vi "spy shoot up.vi"(0 "RPM setting":dbl) -> ()   [LabVIEW 2015]
uses:
  <vilib>/Rock Robotics/WPI/Solenoid/WPI_SolenoidValue.ctl
  <vilib>/Rock Robotics/WPI/CAN/TalonSRX/WPI_CANTalonSRX_APIControlMode.ctl
  <vilib>/Rock Robotics/WPI/Solenoid/WPI_SolenoidSetEnum.vi
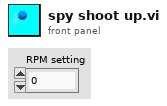
[diagram p1: front panel]
types:
  T1 = typedef "WPI_SolenoidDevRef.ctl" = cluster{"DevStatus":errorcluster, "Pneumatics Control Module":u8, "Forward Solenoid Channel":T2, "Reverse Solenoid Channel":T2}
  T2 = typedef "WPI_SolenoidChannel.ctl" = enum8{"Solenoid 0", "Solenoid 1", "Solenoid 2", "Solenoid 3", "Solenoid 4", "Solenoid 5", "Solenoid 6", "Solenoid 7", "Invalid"}
  T3 = typedef "WPI_MotorControlDeviceRef.ctl" = cluster{"DeviceStatus":errorcluster, "Type":T4, "PWM":cluster{"PWM Channel":T5, "DeadBand":T6}, "CAN":cluster{"Device Number":u8, "Control Mode":T7, "Semaphore":T8, "Max Vout":dbl, "TalonSRX Control Mode":T9}, "Invert":bool}
  T4 = typedef "WPI_MotorControlType.ctl" = enum16{"PWM", "CAN", "CANTalonSRX"}
  T5 = typedef "FPGA_DIOPWMChannel.ctl" = enum8{"PWM 0", "PWM 1", "PWM 2", "PWM 3", "PWM 4", "PWM 5", "PWM 6", "PWM 7", "PWM 8", "PWM 9", "PWM MXP 0", "PWM MXP 1", "PWM MXP 2", "PWM MXP 3", "PWM MXP 4", "PWM MXP 5", "PWM MXP 6", "PWM MXP 7", "PWM MXP 8", "PWM MXP 9", "Invalid"}
  T6 = typedef "WPI_PWMDeadband.ctl" = cluster{"Name":string, "maxPositivePwm":i32, "minPositivePwm":i32, "centerPwm":i32, "maxNegativePwm":i32, "minNegativePwm":i32, "angularRange":u16}
  T7 = typedef "WPI_CANJaguar_ControlMode.ctl" = enum8{"Percent VBus", "Current", "Speed", "Position", "Voltage"}
  T8 = typedef "Semaphore RefNum" = refnum<k1>
  T9 = typedef "WPI_CANTalonSRX_APIControlMode.ctl" = enum8{"Percent VBus", "Speed", "Position", "Slave", "Unchanged / Invalid", "Voltage Compensation", "Current", "Motion Profile"}
  T10 = typedef "WPI_SolenoidValue.ctl" = enum16{"Off", "On", "Forward", "Reverse"}
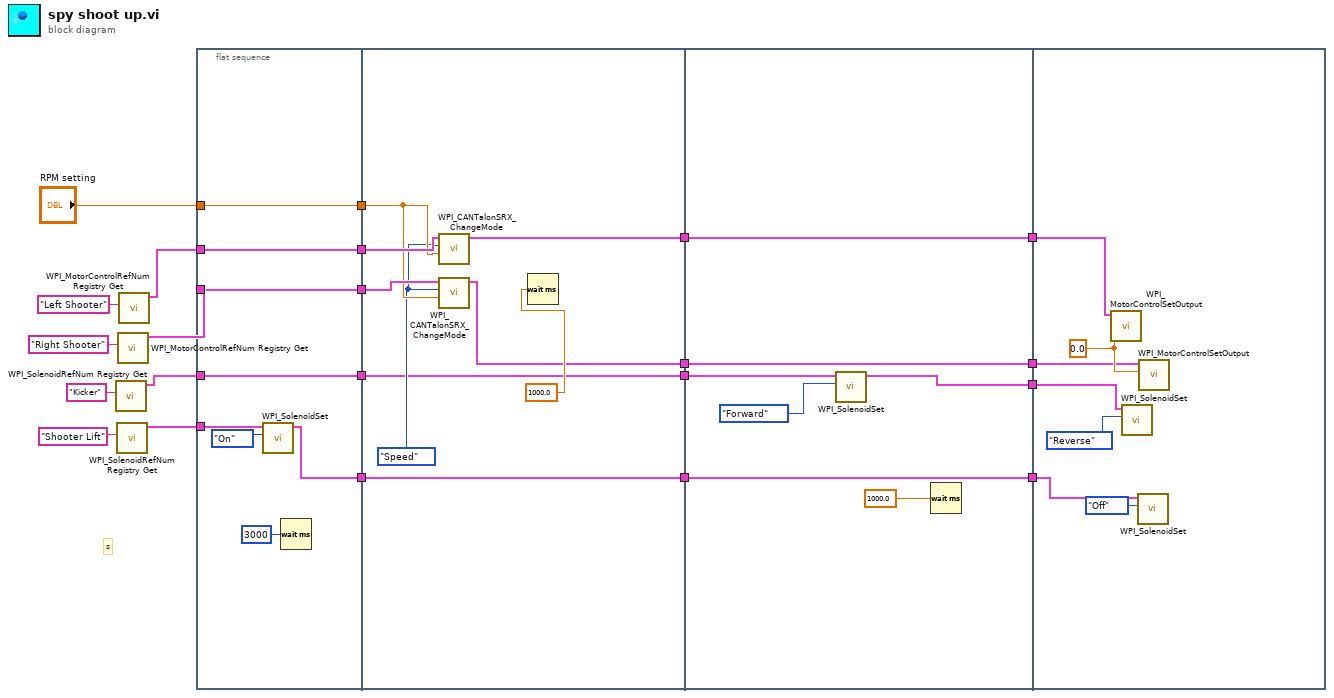
[diagram p0: block diagram]
diagram:
  # "s"
  n1 = call <vilib>:"WPI_SolenoidRefNum Registry Get.vi"("refnum name"="Kicker") -> ("SolenoidDevRef"=w10:T1)  [unwired: 9 in, 1 out]
  n2 = call <vilib>:"WPI_SolenoidRefNum Registry Get.vi"("refnum name"="Shooter Lift") -> ("SolenoidDevRef"=w18:T1)  [unwired: 9 in, 1 out]
  n3 = call <vilib>:"WPI_MotorControlRefNum Registry Get.vi"("refnum name"="Right Shooter") -> ("MotorControlDevRef"=w16:T3)  [unwired: 9 in, 1 out]
  n4 = call <vilib>:"WPI_MotorControlRefNum Registry Get.vi"("refnum name"="Left Shooter") -> ("MotorControlDevRef"=w14:T3)  [unwired: 9 in, 1 out]
  n5 = flat-sequence {
    tunnel: w18 -> [w30]
    tunnel: w16 -> [w28]
    tunnel: [w28] -> w17
    tunnel: w14 -> [w27]
    tunnel: [w27] -> w15
    tunnel: "RPM setting" -> [w26]
    tunnel: [w26] -> w12
    tunnel: [w25] -> w11
    tunnel: w10 -> [w25]
    tunnel: [w24] -> w1
    tunnel: w17 -> [w39]
    tunnel: w15 -> [w38]
    tunnel: w12 -> [w37]
    tunnel: w11 -> [w34]
    tunnel: [w34] -> w9
    tunnel: [w33] -> w7
    tunnel: [w32] -> w5
    tunnel: [w31] -> w2
    tunnel: w1 -> [w31]
    tunnel: w9 -> [w46]
    tunnel: [w43] -> w8
    tunnel: w7 -> [w43]
    tunnel: [w42] -> w6
    tunnel: w5 -> [w42]
    tunnel: [w41] -> w4
    tunnel: [w40] -> w3
    tunnel: w2 -> [w40]
    tunnel: w8 -> [w53]
    tunnel: w6 -> [w51]
    tunnel: w4 -> [w50]
    tunnel: w3 -> [w48]
    frame #0 {
      n6 = call-poly <vilib>:"WPI_SolenoidSet.vi"("Value"=WPI_SolenoidValue."On", "SolenoidDevRef"=w30) -> ("SolenoidDevRef"=w24:T1)  [unwired: 8 in, 1 out]
      n7 = Wait (ms)(milliseconds to wait=u32 3000) -> ()  [unwired: 1 out]
    }
    frame #1 {
      w36 = WPI_CANTalonSRX_APIControlMode."Speed" ("Control Mode")
      n8 = call <vilib>:"WPI_CANTalonSRX_ChangeMode.vi"("Output"=w37, "Control Mode"=w36, "CAN Talon SRX Ref"=w38) -> ("CAN Talon SRX Ref"=w33:T3)  [unwired: 7 in, 1 out]
      n9 = call <vilib>:"WPI_CANTalonSRX_ChangeMode.vi"("Output"=w37, "Control Mode"=w36, "CAN Talon SRX Ref"=w39) -> ("CAN Talon SRX Ref"=w32:T3)  [unwired: 7 in, 1 out]
      n10 = Wait (ms)(milliseconds to wait=1000.0) -> ()  [unwired: 1 out]
    }
    frame #2 {
      n11 = call-poly <vilib>:"WPI_SolenoidSet.vi"("Value"=WPI_SolenoidValue."Forward", "SolenoidDevRef"=w46) -> ("SolenoidDevRef"=w41:T1)  [unwired: 8 in, 1 out]
      n12 = Wait (ms)(milliseconds to wait=1000.0) -> ()  [unwired: 1 out]
    }
    frame #3 {
      w52 = 0.0
      n13 = call <vilib>:"WPI_MotorControlSetOutput.vi"("Output"=w52, "MotorControlDevRef"=w53) -> ()  [unwired: 7 in, 3 out]
      n14 = call-poly <vilib>:"WPI_SolenoidSet.vi"("Value"=WPI_SolenoidValue."Reverse", "SolenoidDevRef"=w50) -> ()  [unwired: 8 in, 2 out]
      n15 = call-poly <vilib>:"WPI_SolenoidSet.vi"("Value"=WPI_SolenoidValue."Off", "SolenoidDevRef"=w48) -> ()  [unwired: 8 in, 2 out]
      n16 = call <vilib>:"WPI_MotorControlSetOutput.vi"("Output"=w52, "MotorControlDevRef"=w51) -> ()  [unwired: 7 in, 3 out]
    }
  }
